vi "CRYReport Part ObjectDeleted Event Callback.vi"(4 "TXTextControl":refnum<k7>, 5 "Event Data":cluster{"ObjectId":i16}, 6 "Control Ref":refnum<k7>, 7 "Event Common Data":T1) -> ()   [LabVIEW 2013]
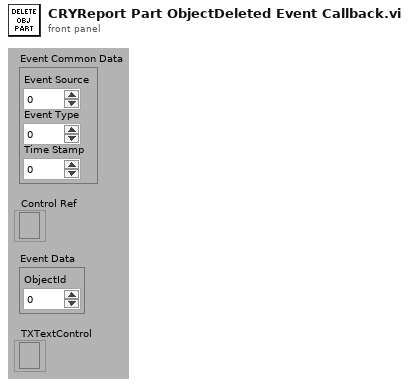
[diagram p1: front panel]
types:
  T1 = cluster{"Event Source":i32, "Event Type":u32, "Time Stamp":u32}
  T2 = cluster{"nID":i16, "sName":string, "pVIRef":refnum<vi>, "pSPRef":refnum<vi>, "sTitle":string, "nIDObject":i16, "nIDV":i16, "nWidth":i16, "nHeight":i16, "bImgChange":bool, "sType":string, "sState":string, "sPosition":string, "sData":string}
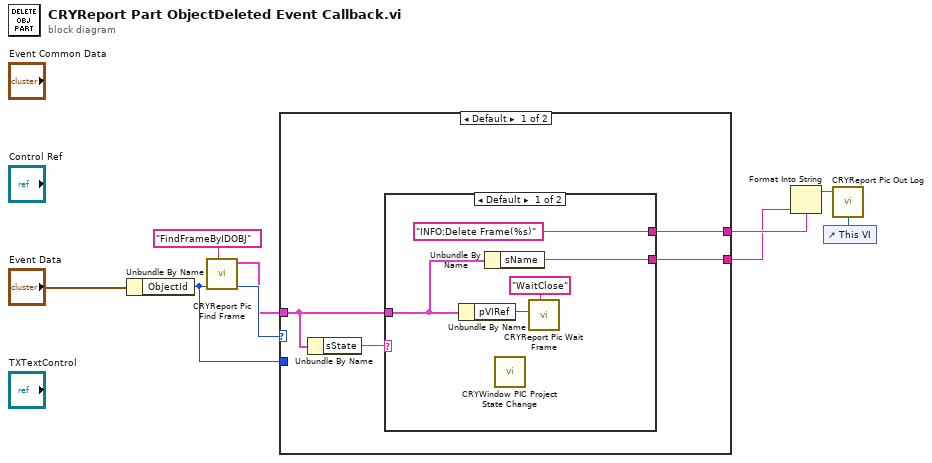
[diagram p0: block diagram]
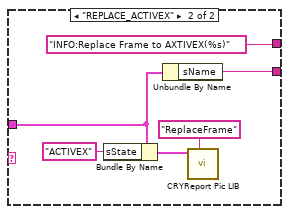
[diagram p2: hidden frame]
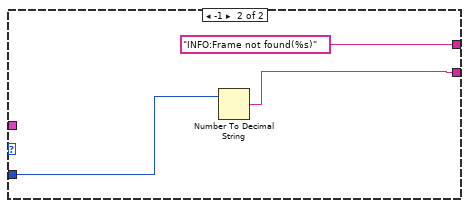
[diagram p3: hidden frame]
diagram:
  n1 = Unbundle By Name("Event Data") -> ("ObjectId"=w6:i16)
  n2 = call "CRYReport Pic Find Frame.vi"("sAction"="FindFrameByIDOBJ", "nData"=w6) -> ("nData_Out"=w8:i32, "cFrame_Out"=w7:T2)  [unwired: 8 in]
  n3 = case shown="Default" w8 {
    tunnel: w7 -> [w12 _]
    tunnel: [w11 "INFO:Frame not found(%s)"] -> w5
    tunnel: w6 -> [_ w26]
    tunnel: [w10 w25] -> w4
    frame Default {
      n4 = Unbundle By Name(w12) -> ("sState"=w13:string)
      n5 = case shown="Default" w13 {
        tunnel: w12 -> [w15 w20]
        tunnel: ["INFO:Delete Frame(%s)" "INFO:Replace Frame to AXTIVEX(%s)"] -> w11
        tunnel: [w14 w19] -> w10
        frame Default {
          n6 = Unbundle By Name(w15) -> ("pVIRef"=w18:refnum<vi>)
          n7 = Unbundle By Name(w15) -> ("sName"=w14:string)
          n8 = call "CRYWindow PIC Project State Change.vi"() -> ()  [unwired: 12 in]
          n9 = call "CRYReport Pic Wait Frame.vi"("sAction"="WaitClose", "vi reference"=w18) -> ()  [unwired: 9 in, 1 out]
        }
        frame "REPLACE_ACTIVEX" {
          n10 = Bundle By Name(cluster=w20, "sState"="ACTIVEX") -> (w23:T2)
          n11 = Unbundle By Name(w20) -> ("sName"=w19:string)
          n12 = call "CRYReport Pic LIB.vi"("sAction"="ReplaceFrame", "cFrame"=w23) -> ()  [unwired: 6 in, 4 out]
        }
      }
    }
    frame -1 {
      n13 = Number To Decimal String(number=w26) -> (decimal integer string=w25:string)  [unwired: 1 in]
    }
  }
  n14 = Format Into String(format string=w5, w4) -> (resulting string=w3:string)  [unwired: 2 in, 1 out]
  n15 = control-ref of="This VI"() -> (w2:refnum<vi>)
  n16 = call "CRYReport Pic Out Log.vi"("vi reference"=w2, "sData"=w3) -> ()  [unwired: 10 in]
